vi "best corr window.vi"(1 "Window":i32(slide)=300 scale=0.0..800.0, 2 "Array 2":dbl[](array[numeric]), 3 "Array 1":dbl[](array[numeric])) -> (0 "corr":dbl)   [LabVIEW 2009]
panel:
  out "corr orig":dbl
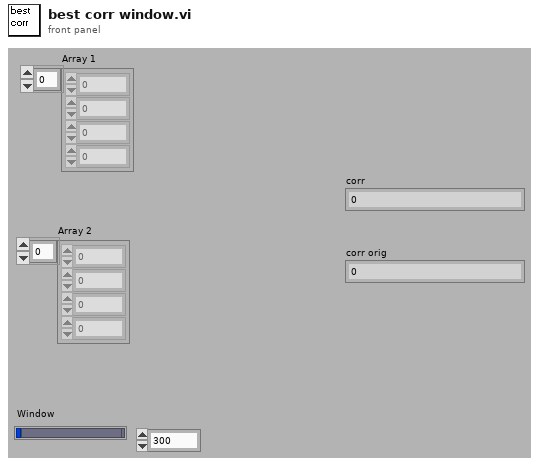
[diagram p1: front panel]
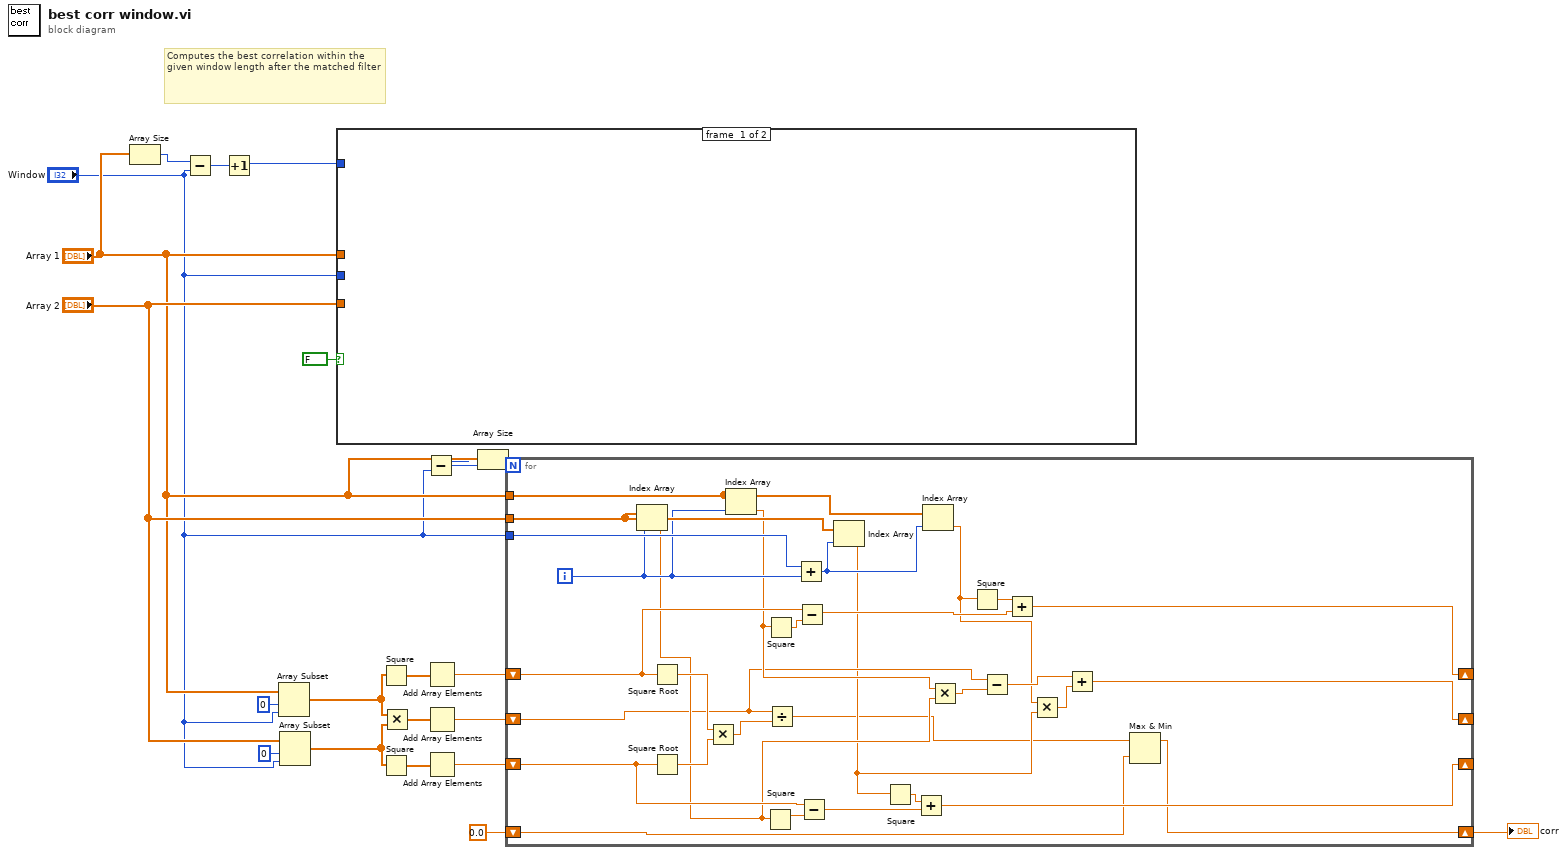
[diagram p0: block diagram]
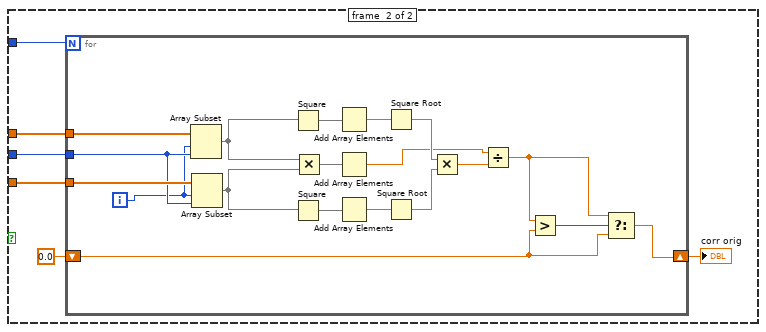
[diagram p2: hidden frame]
diagram:
  # "Computes the best correlation within the given window length after the matched filter"
  n1 = Array Size(array="Array 1") -> (size(s)=w21:i32)
  n2 = Subtract(x=w21, y="Window") -> (x-y=w20:i32)
  n3 = Increment(x=w20) -> (x+1=w19:i32)
  n4 = Array Subset(array="Array 1", index=0, length="Window") -> (w13:dbl[])
  n5 = Array Subset(array="Array 2", index=0, length="Window") -> (w12:dbl[])
  n6 = case shown="True" FALSE {
    tunnel: w19 -> [_ w27]
    tunnel: "Array 2" -> [_ w25]
    tunnel: "Array 1" -> [_ w24]
    tunnel: "Window" -> [_ w23]
    frame #0 {
    }
    frame #1 {
      n7 = for {
        N: w27 -> [_]
        tunnel: w24 -> [w46]
        tunnel: w25 -> [w45]
        tunnel: w23 -> [w44]
        shift-right: [w29] -> w22
        shift-left: 0.0 -> [w28]
        i -> [w43]
        n8 = Array Subset(array=w46, index=w43, length=w44) -> (w41:dbl[])
        n9 = Array Subset(array=w45, index=w43, length=w44) -> (w40:dbl[])
        n10 = Square(x=w41) -> (x^2=w39:dbl[])
        n11 = Square(x=w40) -> (x^2=w38:dbl[])
        n12 = Multiply(x=w41, y=w40) -> (x*y=w42:dbl[])
        n13 = Add Array Elements(numeric array=w39) -> (sum=w37:dbl)
        n14 = Add Array Elements(numeric array=w42) -> (sum=w32:dbl)
        n15 = Add Array Elements(numeric array=w38) -> (sum=w36:dbl)
        n16 = Square Root(x=w37) -> (sqrt(x)=w34:dbl)
        n17 = Square Root(x=w36) -> (sqrt(x)=w35:dbl)
        n18 = Multiply(x=w34, y=w35) -> (x*y=w33:dbl)
        n19 = Divide(x=w32, y=w33) -> (x/y=w30:dbl)
        n20 = Greater?(x=w30, y=w28) -> (0:w31:bool)
        n21 = Select(t=w30, s=w31, f=w28) -> (s? t:f=w29:dbl)
      }
      "corr orig" <- w22
    }
  }
  n22 = Square(x=w13) -> (x^2=w15:dbl[])
  n23 = Square(x=w12) -> (x^2=w14:dbl[])
  n24 = Multiply(x=w13, y=w12) -> (x*y=w16:dbl[])
  n25 = Add Array Elements(numeric array=w15) -> (sum=w11:dbl)
  n26 = Add Array Elements(numeric array=w16) -> (sum=w10:dbl)
  n27 = Add Array Elements(numeric array=w14) -> (sum=w9:dbl)
  n28 = Array Size(array="Array 1") -> (size(s)=w6:i32)
  n29 = Subtract(x=w6, y="Window") -> (x-y=w4:i32)
  n30 = for {
    N: w4 -> [_]
    tunnel: "Array 1" -> [w71]
    tunnel: "Array 2" -> [w70]
    tunnel: "Window" -> [w76]
    shift-right: [w60] -> _
    shift-left: w11 -> [w68]
    shift-right: [w50] -> _
    shift-left: w10 -> [w55]
    shift-right: [w59] -> _
    shift-left: w9 -> [w65]
    shift-right: [w47] -> w2
    shift-left: 0.0 -> [w49]
    i -> [w69]
    n31 = Index Array(array=w70, index=w69) -> (element=w57:dbl)
    n32 = Square Root(x=w68) -> (sqrt(x)=w75:dbl)
    n33 = Square Root(x=w65) -> (sqrt(x)=w74:dbl)
    n34 = Multiply(x=w75, y=w74) -> (x*y=w73:dbl)
    n35 = Index Array(array=w71, index=w69) -> (element=w58:dbl)
    n36 = Square(x=w57) -> (x^2=w66:dbl)
    n37 = Square(x=w58) -> (x^2=w67:dbl)
    n38 = Divide(x=w55, y=w73) -> (x/y=w48:dbl)
    n39 = Add(x=w76, y=w69) -> (x+y=w72:i32)
    n40 = Subtract(x=w68, y=w67) -> (x-y=w63:dbl)
    n41 = Subtract(x=w65, y=w66) -> (x-y=w62:dbl)
    n42 = Index Array(array=w70, index=w72) -> (element=w51:dbl)
    n43 = Square(x=w51) -> (x^2=w61:dbl)
    n44 = Add(x=w61, y=w62) -> (x+y=w59:dbl)
    n45 = Index Array(array=w71, index=w72) -> (element=w52:dbl)
    n46 = Multiply(x=w58, y=w57) -> (x*y=w56:dbl)
    n47 = Square(x=w52) -> (x^2=w64:dbl)
    n48 = Subtract(x=w55, y=w56) -> (x-y=w53:dbl)
    n49 = Add(x=w64, y=w63) -> (x+y=w60:dbl)
    n50 = Multiply(x=w52, y=w51) -> (x*y=w54:dbl)
    n51 = Add(x=w53, y=w54) -> (x+y=w50:dbl)
    n52 = Max & Min(x=w48, y=w49) -> (max(x,y)=w47:dbl)  [unwired: 1 out]
  }
  "corr" <- w2
